vi "Set Dev Panel.vi"(10 "Dev Panel":refnum<class "Dev Panel.lvclass">, 11 "Dev Actor in":refnum<class "Dev Actor.lvclass">) -> (3 "Dev Actor out":refnum<class "Dev Actor.lvclass">)   [LabVIEW 2021]
uses:
  Dev Actor.lvclass
  Dev Panel/Dev Panel.lvclass
  Dev Actor.lvclass/Dev Actor.ctl
  C:/Program Files/National Instruments/LabVIEW 2021/vi.lib/jettl/jettl/Actor/Actor/Actor.lvclass
  C:/Program Files/National Instruments/LabVIEW 2021/vi.lib/jettl/jettl/Actor/Msgs/Create/Create/Create.lvclass
  C:/Program Files/National Instruments/LabVIEW 2021/vi.lib/jettl/jettl/Actor/Msgs/Last Ack/Last Ack/Last Ack.lvclass
  C:/Program Files/National Instruments/LabVIEW 2021/vi.lib/jettl/jettl/Actor/Msgs/Merge Error/Merge Error/Merge Error.lvclass
  C:/Program Files/National Instruments/LabVIEW 2021/vi.lib/jettl/jettl/Actor/Msgs/Override Error/Override Error/Override Error.lvclass
  C:/Program Files/National Instruments/LabVIEW 2021/vi.lib/jettl/jettl/Actor/Msgs/Teardown/Teardown/Teardown.lvclass
  C:/git/Dev-Actor/src/Dev Actor/Dev Actor/Dev Actor.lvclass
  C:/git/Dev-Actor/src/Helper Loop/Msgs/Helper Loop Create/Helper Loop Create/Helper Loop Create.lvclass
  C:/git/Dev-Actor/src/Helper Loop/Helper Loop/Helper Loop.lvclass
  C:/git/Dev-Actor/src/Msgs/Pop Up/Pop Up/Pop Up.lvclass
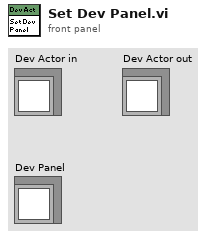
[diagram p1: front panel]
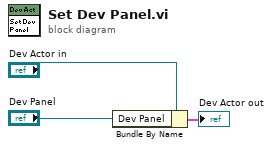
[diagram p0: block diagram]
diagram:
  n1 = Bundle By Name(cluster="Dev Actor in", "Dev Panel"="Dev Panel") -> (→"Dev Actor out":cluster{})
